vi "Read Key (Raw).vi"(7 "Section Name":string, 8 "error in (no error)":errorcluster, 10 "Key Name":string, 11 "Config in":refnum<class "LabVIEW-Config.lvclass">) -> (0 "error out":errorcluster, 1 "Content":string, 2 "Key Found?":bool, 3 "Config out":refnum<class "LabVIEW-Config.lvclass">)   [LabVIEW 2017, in "LabVIEW-Config.lvlib" / "LabVIEW-Config.lvclass"]
uses:
  LabVIEW-Config.lvclass
  LabVIEW-Config.lvclass/LabVIEW-Config.ctl
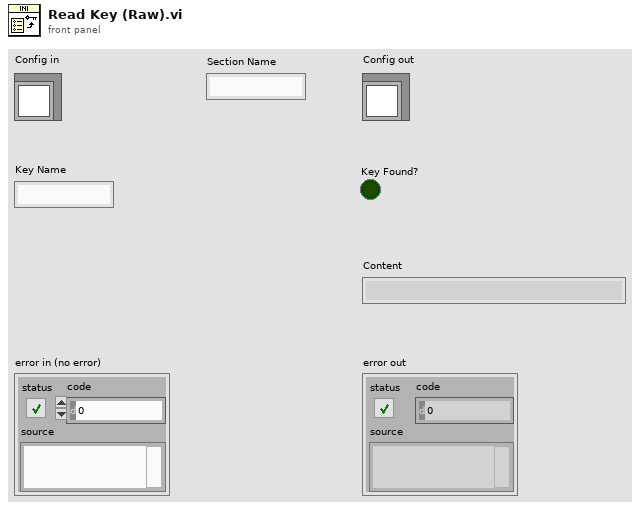
[diagram p1: front panel]
types:
  T1 = typedef "LabVIEW-Config.lvlib/LabVIEW-Config.lvclass/KeyInfo.ctl" = cluster{"Key Indexes":cluster{"Indexes":i32[]}[], "Session Found?":bool, "Key found?":bool, "Session Index":i32}
  T2 = typedef "LabVIEW-Config.lvlib/LabVIEW-Config.lvclass/LineToken.ctl" = enum8{"comment", "section", "key", "more"}
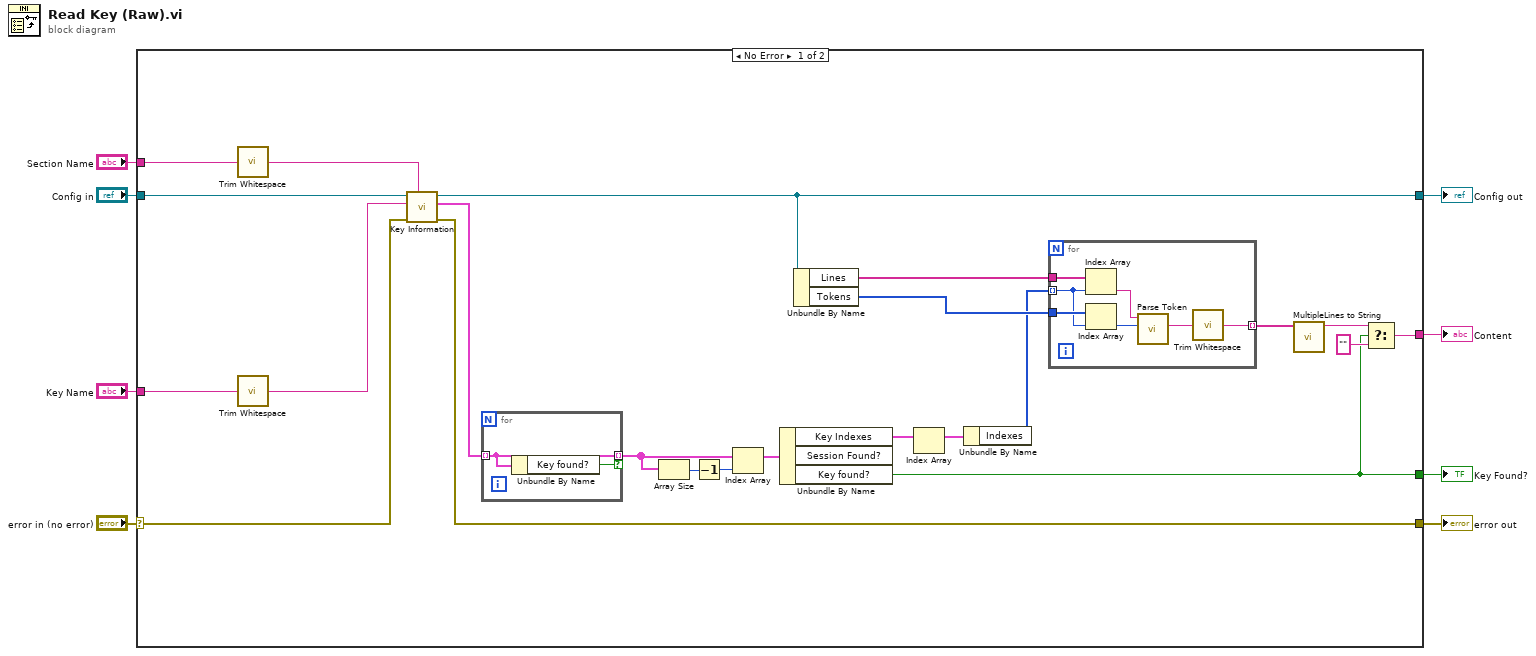
[diagram p0: block diagram]
diagram:
  n1 = case shown="No Error" "error in (no error)" {
    selector: "error in (no error)" -> [w25 w42]
    tunnel: "Config in" -> [w28 w41]
    tunnel: [w24 w42] -> w7
    tunnel: [w22 w41] -> w5
    tunnel: "Section Name" -> [w27 _]
    tunnel: "Key Name" -> [w26 _]
    tunnel: [w30 _] -> w2
    tunnel: [w23 _] -> w1
    frame No Error {
      n2 = call <vilib>:"Trim Whitespace.vi"("string"=w27) -> ("trimmed string"=w17:string)  [unwired: 1 in]
      n3 = call <vilib>:"Trim Whitespace.vi"("string"=w26) -> ("trimmed string"=w16:string)  [unwired: 1 in]
      n4 = call "Key Information.vi"("Section Name"=w17, "error in (no error)"=w25, "Key Name"=w16, "Config in"=w28) -> ("error out"=w24:errorcluster, "Key Information"=w12:T1[], "Config out"=w22:refnum<class "LabVIEW-Config.lvclass">)  [unwired: 5 in]
      n5 = for {
        tunnel: w12 -> [w33] mode=indexing
        tunnel: [w33] -> w11 mode=indexing if=w32
        n6 = Unbundle By Name(w33) -> ("Key found?"=w32:bool)
      }
      n7 = Array Size(array=w11) -> (size(s)=w14:i32)
      n8 = Decrement(x=w14) -> (x-1=w13:i32)
      n9 = Index Array(array=w11, index=w13) -> (element=w15:T1)
      n10 = Unbundle By Name(w15) -> ("Key Indexes"=w20:cluster{"Indexes":i32[]}[], "Key found?"=w23:bool)  [unwired: 1 out]
      n11 = Unbundle By Name(w22) -> ("Lines"=w21:string[], "Tokens"=w19:T2[])
      n12 = Index Array(array=w20) -> (element=w10:cluster{"Indexes":i32[]})  [unwired: 1 in]
      n13 = Unbundle By Name(w10) -> ("Indexes"=w9:i32[])
      n14 = for {
        tunnel: w21 -> [w40]
        tunnel: w9 -> [w37] mode=indexing
        tunnel: w19 -> [w38]
        tunnel: [w34] -> w18 mode=indexing
        n15 = Index Array(array=w40, index=w37) -> (element=w39:string)
        n16 = Index Array(array=w38, index=w37) -> (element=w36:T2)
        n17 = call "Parse Token.vi"("Token"=w36, "Line"=w39) -> ("Value"=w35:string)  [unwired: 8 in, 1 out]
        n18 = call <vilib>:"Trim Whitespace.vi"("string"=w35) -> ("trimmed string"=w34:string)  [unwired: 1 in]
      }
      n19 = call "MultipleLines to String.vi"("Array"=w18) -> ("String"=w29:string)  [unwired: 10 in]
      n20 = Select(t=w29, s=w23, f="") -> (s? t:f=w30:string)
    }
    frame Error {
    }
  }
  "error out" <- w7
  "Config out" <- w5
  "Key Found?" <- w1
  "Content" <- w2
